vi "Add Routing Channel RTM.vi"(8 "error in (no error)":errorcluster, 11 "Node Ptr":u64 format="%.0x") -> (0 "error out":errorcluster)   [LabVIEW 2020, in "Routing and Faulting System Explorer.lvlib"]
uses:
  Routing and Faulting System Explorer.lvlib
  Shared/Constants.vi
  Scripting/Routing and Faulting Scripting.lvlib
  Shared/Routing and Faulting Shared.lvlib
  <vilib>/NI VeriStand/Custom Device Tools/Custom Device Utility Library/Custom Device Utility Library.lvlib
panel:
  in  "Tag":string
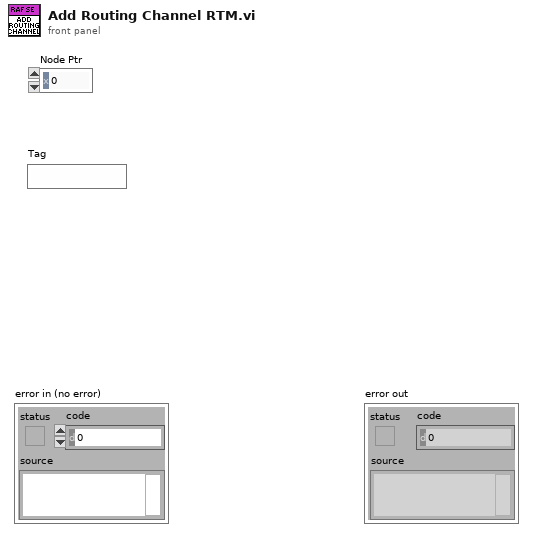
[diagram p1: front panel]
types:
  T1 = typedef "Custom Device API.lvlib/Custom Device Item Ref.ctl" = u64
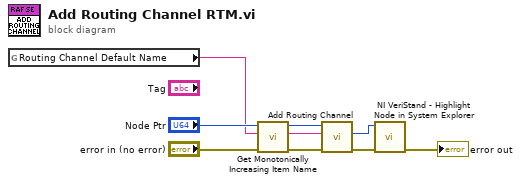
[diagram p0: block diagram]
diagram:
  n1 = global read "Constants.vi" "Routing Channel Default Name"() -> (w4:string)
  n2 = call "Get Monotonically Increasing Item Name.vi"("error in (no error)"="error in (no error)", "Desired Name"=w4, "Section Ptr"="Node Ptr") -> ("error out"=w6:errorcluster, "New Item Name"=w5:string, "Section Ptr out"=w7:T1)  [unwired: 6 in]
  n3 = call "Add Routing Channel.vi"("error in"=w6, "channel name"=w5, "routing channels in"=w7) -> ("error out"=w3:errorcluster, "routing channel"=w1:T1)  [unwired: 6 in, 1 out]
  n4 = call <vilib>:"NI VeriStand - Highlight Node in System Explorer.vi"("error in (no error)"=w3, "Item Ref in"=w1) -> ("error out"=→"error out":errorcluster)  [unwired: 8 in, 1 out]
